vi "Selection Y-axis.vi"(8 "error in (no error)":errorcluster, 9 "Config":T1={"Selection"={"caption"="", "Validaty Threshold"=2, "Color"=6618880, "Start Coords"={"Horizental"=0, "Vertical"=0}}}, 10 "GrphChrt Refnum":refnum<vi>, 11 "picture":picture) -> (0 "error out":errorcluster, 1 "Output Valid":bool, 2 "Y2":dbl, 3 "Y1":dbl)   [LabVIEW 2019, in "Graph Tools.lvlib"]
uses:
  Graph Tools.lvlib
  [Selection] Config.ctl
  <vilib>/Utility/miscctls.llb/LVPoint32TypeDef.ctl
  Selection VIs/controls/MarkerOptions.ctl
  Selection VIs/controls/markerType.ctl
  <vilib>/Utility/inputDevices.llb/mouseAcquire.vi
  <vilib>/Utility/inputDevices.llb/closeMouse.vi
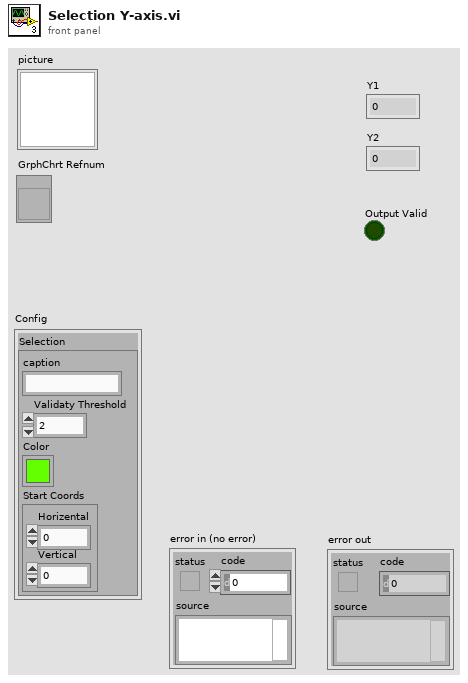
[diagram p1: front panel]
types:
  T1 = typedef "Graph Tools.lvlib/[Selection] Config.ctl" = cluster{"Selection":cluster{"caption":string, "Validaty Threshold":i32, "Color":u32, "Start Coords":T2}}
  T2 = typedef "LVPoint32TypeDef.ctl" = cluster{"Horizental":i32, "Vertical":i32}
  T3 = typedef "MarkerOptions.ctl" = cluster{"Color":u32, "pen":cluster{"Width":u16, "Style":enum32{"Solid", "Dash", "Dot", "DashDot", "DashDotDot"}}, "font":cluster{"Font Name":string, "Size":i16, "Strikeout?":bool, "Italic?":bool, "Underline?":bool, "Outline?":bool, "Shadow?":bool, "Bold?":bool, "FontColor":u32}, "caption":string}
  T4 = typedef "markerType.ctl" = enum16{"point", "arrow", "horiz", "vert", "vert range", "horiz range", "box"}
  T5 = cluster{"Horizontal":i32, "Vertical":i32, "Scrolling":i32}
  T6 = typedef "LVRectTypeDef.ctl" = cluster{"Left":i16, "Top":i16, "Right":i16, "Bottom":i16}
  T7 = cluster{"button 1":bool, "button 2":bool, "button 3":bool, "button 4":bool}
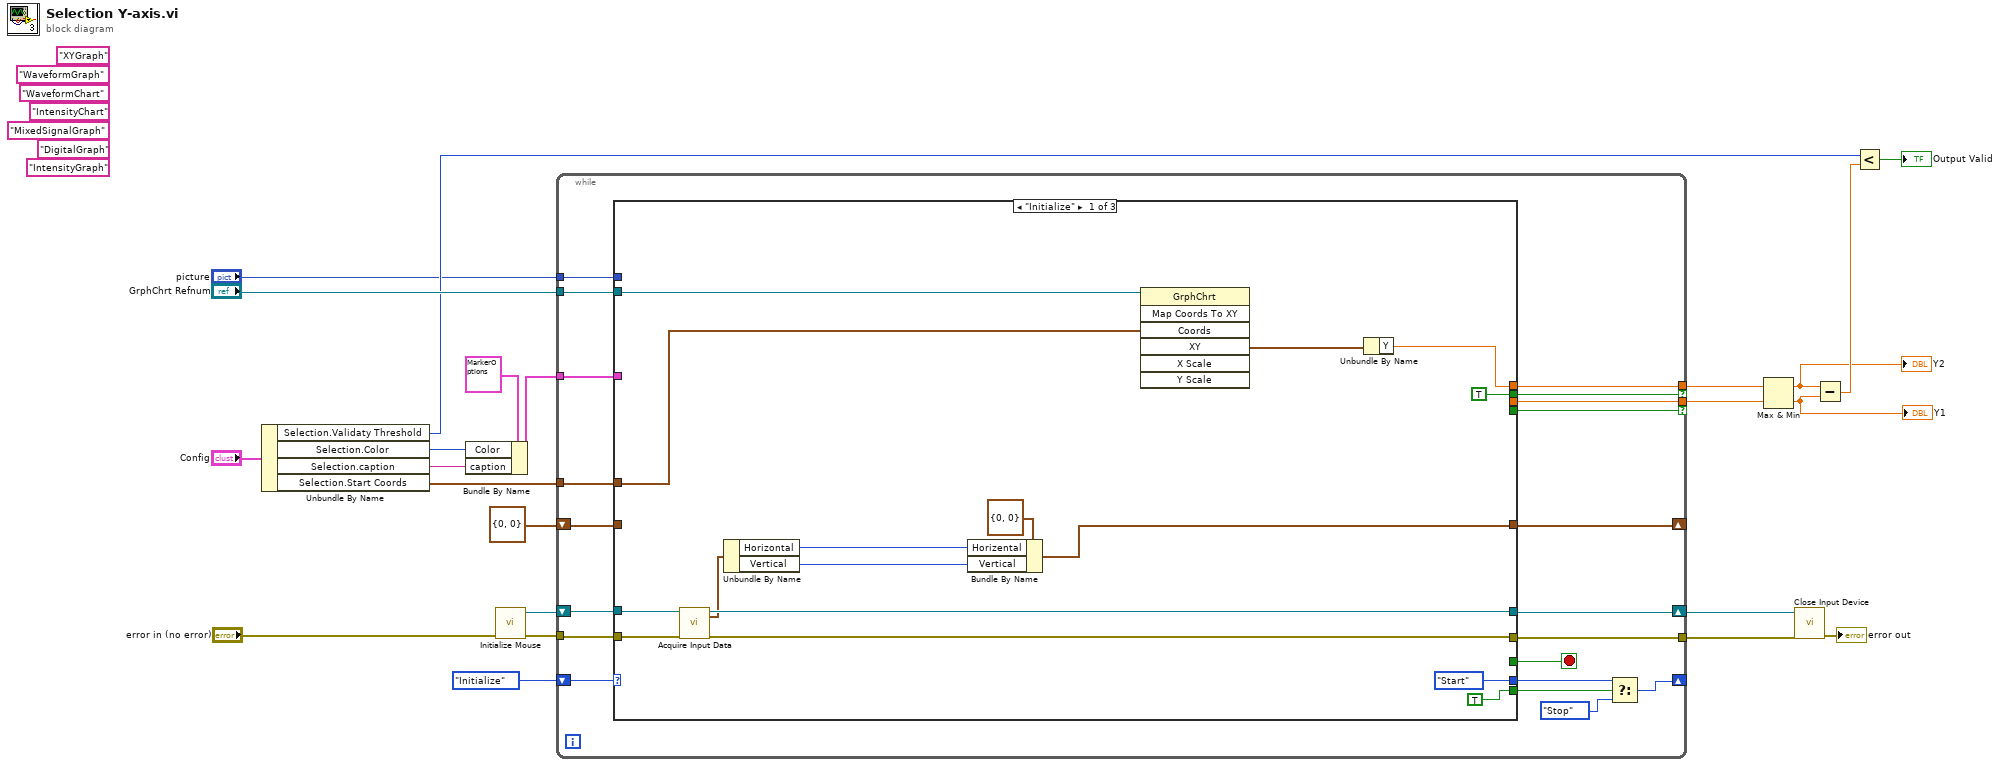
[diagram p0: block diagram]
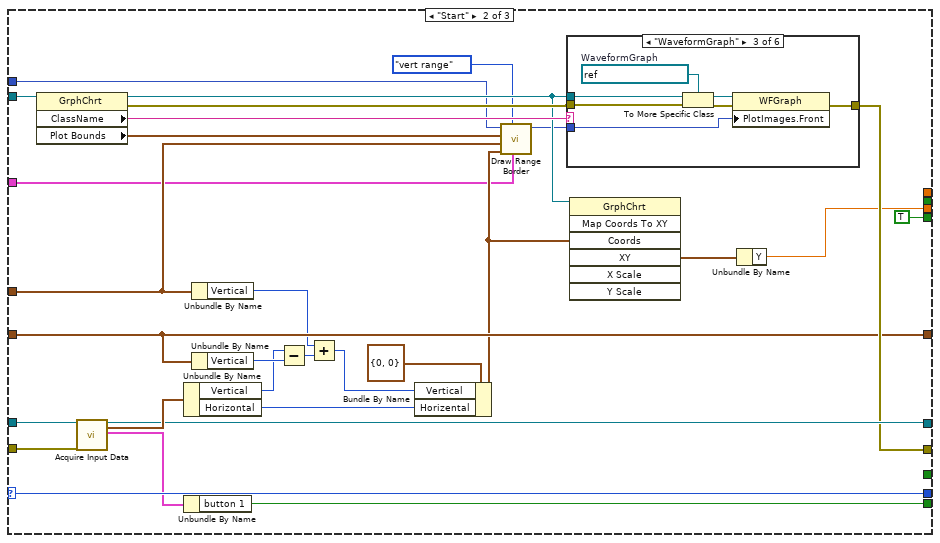
[diagram p2: hidden frame]
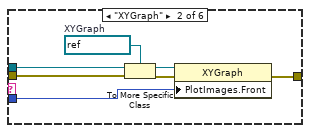
[diagram p4: hidden frame]
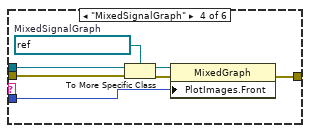
[diagram p5: hidden frame]
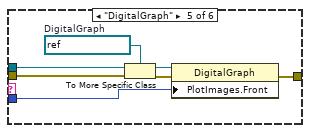
[diagram p6: hidden frame]
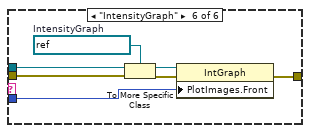
[diagram p7: hidden frame]
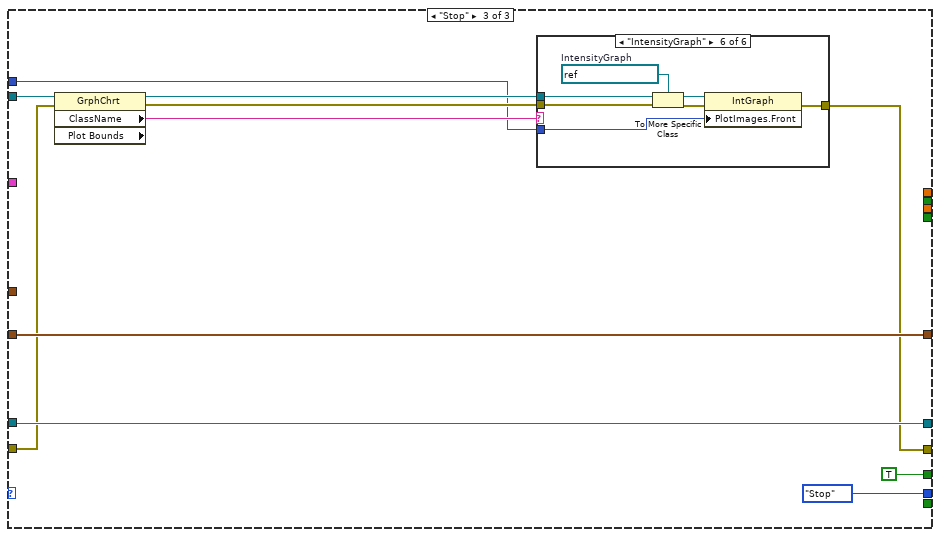
[diagram p8: hidden frame]
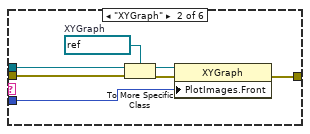
[diagram p10: hidden frame]
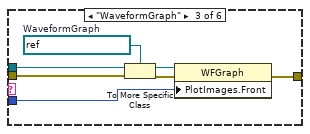
[diagram p11: hidden frame]
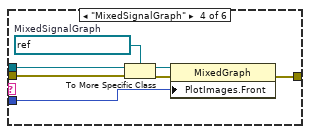
[diagram p12: hidden frame]
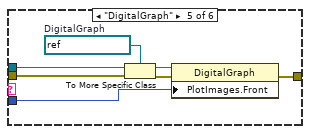
[diagram p13: hidden frame]
diagram:
  (unwired) "IntensityGraph" ("Class Name 4")
  (unwired) "DigitalGraph" ("Class Name 3")
  (unwired) "MixedSignalGraph" ("Class Name 2")
  (unwired) "XYGraph" ("Class Name 2")
  (unwired) "IntensityChart" ("Class Name 3")
  (unwired) "WaveformChart" ("Class Name 4")
  (unwired) "WaveformGraph" ("Class Name 5")
  n1 = Unbundle By Name("Config") -> ("Selection.Validaty Threshold"=w8:i32, "Selection.Color"=w15:u32, "Selection.caption"=w14:string, "Selection.Start Coords"=w6:T2)
  n2 = Bundle By Name(cluster=T3 {"Color"=16723218, "pen"={"Width"=2, "Style"=enum."Solid"}, "font"={"Font Name"="Arial", "Size"=16, "Strikeout?"=FALSE, "Italic?"=FALSE, "Underline?"=FALSE, "Outline?"=FALSE, "Shadow?"=FALSE, "Bold?"=FALSE, "FontColor"=0}, "caption"=""} ("Marker Options"), "Color"=w15, "caption"=w14) -> (w16:T3)
  n3 = call <vilib>:"Initialize Mouse.vi"("error in (no error)"="error in (no error)") -> ("error out"=w20:errorcluster, "device ID"=w23:refnum<k1>)  [unwired: 9 in]
  n4 = while {
    tunnel: [w32] -> w21
    tunnel: w20 -> [w35]
    shift-right: [w39] -> _
    shift-left: enum16{"Initialize", "Start", "Stop"}."Initialize" -> [w41]
    tunnel: "GrphChrt Refnum" -> [w38]
    tunnel: w16 -> [w37]
    shift-right: [w33] -> w22
    shift-left: w23 -> [w36]
    shift-right: [w31] -> _
    shift-left: T2 {"Horizental"=0, "Vertical"=0} ("Start Coords") -> [w30]
    tunnel: w6 -> [w29]
    tunnel: "picture" -> [w28]
    tunnel: [w27] -> w2 if=w26
    tunnel: [w24] -> w1 if=w25
    stop <- w43 stop-if-true
    n5 = case shown="\"Initialize\"" w41 {
      selector: w41 -> [_ w89 _]
      tunnel: [enum16{"Initialize", "Start", "Stop"}."Start" ("f") w89 enum16{"Initialize", "Start", "Stop"}."Stop" ("f")] -> w40
      tunnel: [_ _ TRUE] -> w43
      tunnel: w38 -> [w48 w78 w132]
      tunnel: w37 -> [_ w62 _]
      tunnel: w36 -> [w56 w86 w134]
      tunnel: w35 -> [w54 w85 w126]
      tunnel: [TRUE ("button 1") w84 _] -> w34
      tunnel: [w55 w83 w134] -> w33
      tunnel: [w53 w80 w127] -> w32
      tunnel: [_ TRUE _] -> w25
      tunnel: [TRUE _ _] -> w26
      tunnel: [w49 w74 w133] -> w31
      tunnel: w30 -> [_ w74 w133]
      tunnel: w29 -> [w46 w63 _]
      tunnel: w28 -> [_ w68 w128]
      tunnel: [w44 _ _] -> w27
      tunnel: [_ w60 _] -> w24
      frame "Initialize" {
        n6 = call-poly <vilib>:"Acquire Input Data.vi"("device ID"=w56, "error in (no error)"=w54) -> ("device ID"=w55:refnum<k1>, "axis info"=w52:T5, "error out"=w53:errorcluster)  [unwired: 14 in, 1 out]
        n7 = Unbundle By Name(w52) -> ("Horizontal"=w47:i32, "Vertical"=w51:i32)
        n8 = Bundle By Name(cluster=T2 {"Horizental"=0, "Vertical"=0} ("Start Coords"), "Horizental"=w47, "Vertical"=w51) -> (w49:T2)
        n9 = invoke class="GrphChrt" method="Map Coords To XY"(reference=w48, "Coords"=w46) -> ("XY"=w45:cluster{"X":dbl, "Y":dbl})  [unwired: 5 in, 6 out]
        n10 = Unbundle By Name(w45) -> ("Y"=w44:dbl)
      }
      frame "Start" {
        n11 = property class="GrphChrt"(reference=w78) -> (reference out=w76:refnum<vi>, error out=w81:errorcluster, "ClassName"=w79:string, "Plot Bounds"=w65:T6)  [unwired: 1 in]
        n12 = call-poly <vilib>:"Acquire Input Data.vi"("device ID"=w86, "error in (no error)"=w85) -> ("device ID"=w83:refnum<k1>, "axis info"=w88:T5, "button info"=w87:T7)  [unwired: 14 in, 1 out]
        n13 = Unbundle By Name(w88) -> ("Vertical"=w72:i32, "Horizontal"=w77:i32)
        n14 = Unbundle By Name(w87) -> ("button 1"=w84:bool)
        n15 = Unbundle By Name(w63) -> ("Vertical"=w69:i32)
        n16 = Unbundle By Name(w74) -> ("Vertical"=w73:i32)
        n17 = Subtract(x=w72, y=w73) -> (x-y=w71:i32)
        n18 = Add(x=w69, y=w71) -> (x+y=w70:i32)
        n19 = Bundle By Name(cluster=T2 {"Horizental"=0, "Vertical"=0} ("Start Coords"), "Vertical"=w70, "Horizental"=w77) -> (w64:T2)
        n20 = call "Draw Range Border.vi"("Marker Options"=w62, "Type"=markerType."vert range", "end Coords"=w64, "Start Coords"=w63, "Plot Bounds"=w65, "picture"=w68) -> ("new picture"=w67:picture)  [unwired: 5 in]
        n21 = case shown="\"WaveformGraph\"" w79 {
          tunnel: w76 -> [_ w97 w104 w111 w118 w125]
          tunnel: w81 -> [w90 w95 w102 w106 w113 w120]
          tunnel: w67 -> [_ w93 w98 w105 w112 w119]
          tunnel: [w90 w91 w100 w108 w115 w122] -> w80
          frame Default {
          }
          frame "XYGraph" {
            w96 = refnum<vi> refnum  # XYGraph
            n22 = To More Specific Class(target class=w96, reference=w97, error in=w95) -> (specific class reference=w94:refnum<vi>, error out=w92:errorcluster)
            n23 = property class="XYGraph"(reference=w94, error in=w92, "PlotImages.Front"=w93) -> (error out=w91:errorcluster)  [unwired: 1 out]
          }
          frame "WaveformGraph" {
            w103 = refnum<vi> refnum  # WaveformGraph
            n24 = To More Specific Class(target class=w103, reference=w104, error in=w102) -> (specific class reference=w101:refnum<vi>, error out=w99:errorcluster)
            n25 = property class="WFGraph"(reference=w101, error in=w99, "PlotImages.Front"=w98) -> (error out=w100:errorcluster)  [unwired: 1 out]
          }
          frame "MixedSignalGraph" {
            w110 = refnum<vi> refnum  # MixedSignalGraph
            n26 = To More Specific Class(target class=w110, reference=w111, error in=w106) -> (specific class reference=w109:refnum<vi>, error out=w107:errorcluster)
            n27 = property class="MixedGraph"(reference=w109, error in=w107, "PlotImages.Front"=w105) -> (error out=w108:errorcluster)  [unwired: 1 out]
          }
          frame "DigitalGraph" {
            w117 = refnum<vi> refnum  # DigitalGraph
            n28 = To More Specific Class(target class=w117, reference=w118, error in=w113) -> (specific class reference=w116:refnum<vi>, error out=w114:errorcluster)
            n29 = property class="DigitalGraph"(reference=w116, error in=w114, "PlotImages.Front"=w112) -> (error out=w115:errorcluster)  [unwired: 1 out]
          }
          frame "IntensityGraph" {
            w124 = refnum<vi> refnum  # IntensityGraph
            n30 = To More Specific Class(target class=w124, reference=w125, error in=w120) -> (specific class reference=w123:refnum<vi>, error out=w121:errorcluster)
            n31 = property class="IntGraph"(reference=w123, error in=w121, "PlotImages.Front"=w119) -> (error out=w122:errorcluster)  [unwired: 1 out]
          }
        }
        n32 = invoke class="GrphChrt" method="Map Coords To XY"(reference=w76, "Coords"=w64) -> ("XY"=w61:cluster{"X":dbl, "Y":dbl})  [unwired: 5 in, 6 out]
        n33 = Unbundle By Name(w61) -> ("Y"=w60:dbl)
      }
      frame "Stop" {
        n34 = property class="GrphChrt" props=["ClassName", "Plot Bounds"](reference=w132, error in=w126) -> (reference out=w131:refnum<vi>, error out=w130:errorcluster, "ClassName"=w129:string)  [unwired: 1 out]
        n35 = case shown="\"IntensityGraph\"" w129 {
          tunnel: w131 -> [_ w144 w151 w158 w165 w172]
          tunnel: w130 -> [w137 w142 w149 w153 w160 w167]
          tunnel: w128 -> [_ w140 w145 w152 w159 w166]
          tunnel: [w137 w138 w147 w155 w162 w169] -> w127
          frame Default {
          }
          frame "XYGraph" {
            w143 = refnum<vi> refnum  # XYGraph
            n36 = To More Specific Class(target class=w143, reference=w144, error in=w142) -> (specific class reference=w141:refnum<vi>, error out=w139:errorcluster)
            n37 = property class="XYGraph"(reference=w141, error in=w139, "PlotImages.Front"=w140) -> (error out=w138:errorcluster)  [unwired: 1 out]
          }
          frame "WaveformGraph" {
            w150 = refnum<vi> refnum  # WaveformGraph
            n38 = To More Specific Class(target class=w150, reference=w151, error in=w149) -> (specific class reference=w148:refnum<vi>, error out=w146:errorcluster)
            n39 = property class="WFGraph"(reference=w148, error in=w146, "PlotImages.Front"=w145) -> (error out=w147:errorcluster)  [unwired: 1 out]
          }
          frame "MixedSignalGraph" {
            w157 = refnum<vi> refnum  # MixedSignalGraph
            n40 = To More Specific Class(target class=w157, reference=w158, error in=w153) -> (specific class reference=w156:refnum<vi>, error out=w154:errorcluster)
            n41 = property class="MixedGraph"(reference=w156, error in=w154, "PlotImages.Front"=w152) -> (error out=w155:errorcluster)  [unwired: 1 out]
          }
          frame "DigitalGraph" {
            w164 = refnum<vi> refnum  # DigitalGraph
            n42 = To More Specific Class(target class=w164, reference=w165, error in=w160) -> (specific class reference=w163:refnum<vi>, error out=w161:errorcluster)
            n43 = property class="DigitalGraph"(reference=w163, error in=w161, "PlotImages.Front"=w159) -> (error out=w162:errorcluster)  [unwired: 1 out]
          }
          frame "IntensityGraph" {
            w171 = refnum<vi> refnum  # IntensityGraph
            n44 = To More Specific Class(target class=w171, reference=w172, error in=w167) -> (specific class reference=w170:refnum<vi>, error out=w168:errorcluster)
            n45 = property class="IntGraph"(reference=w170, error in=w168, "PlotImages.Front"=w166) -> (error out=w169:errorcluster)  [unwired: 1 out]
          }
        }
      }
    }
    n46 = Select(t=w40, s=w34, f=enum16{"Initialize", "Start", "Stop"}."Stop") -> (s? t:f=w39:enum16{"Initialize", "Start", "Stop"})
  }
  n47 = Max & Min(x=w2, y=w1) -> (max(x,y)=w5:dbl, min(x,y)=w4:dbl)
  "Y2" <- w5
  "Y1" <- w4
  n48 = call-poly <vilib>:"Close Input Device.vi"("error in (no error)"=w21, "device ID"=w22) -> ("error out"=→"error out":errorcluster)  [unwired: 8 in]
  n49 = Subtract(x=w5, y=w4) -> (x-y=w10:dbl)
  n50 = Less?(x=w8, y=w10) -> (x < y?=→"Output Valid":bool)
